vi "Write to Hardware.vi"(8 "error in":errorcluster, 10 "Values in":dbl[](array[numeric]), 11 "Ballard ARINC-429 Execution Unit in":refnum<class "Ballard ARINC-429 Execution Unit.lvclass">) -> (0 "error out":errorcluster, 2 "Values out":dbl[](array[numeric]), 3 "Ballard ARINC-429 Execution Unit out":refnum<class "Ballard ARINC-429 Execution Unit.lvclass">)   [LabVIEW 2020, in "Ballard ARINC 429 Engine.lvlib" / "Implementation.lvlib" / "Ballard ARINC-429 Execution Unit.lvclass"]
uses:
  Ballard ARINC-429 Execution Unit.lvclass
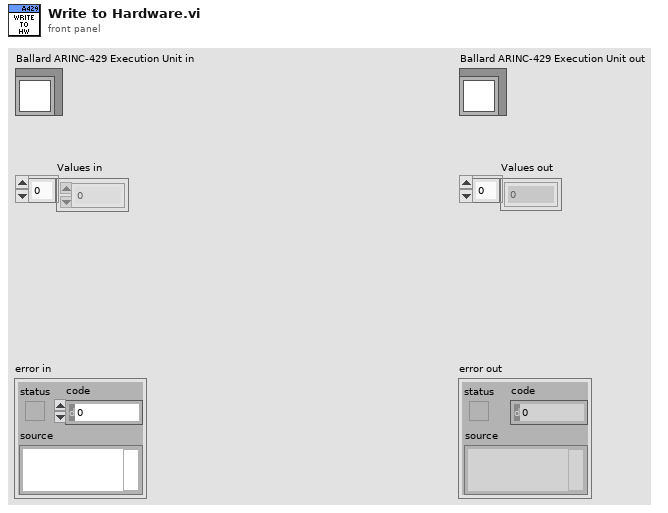
[diagram p1: front panel]
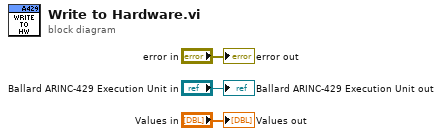
[diagram p0: block diagram]
diagram:
  "error out" <- "error in"
  "Ballard ARINC-429 Execution Unit out" <- "Ballard ARINC-429 Execution Unit in"
  "Values out" <- "Values in"
